vi "Query Active Channel.vi"(8 "error in (no error)":errorcluster, 11 "VISA resource name":refnum<visa-resource-name>) -> (0 "error out":errorcluster, 2 "Active Channel":u16(ring) items=["", "Channel 1", "Channel 2"], 3 "VISA resource name out":refnum<visa-resource-name>)   [LabVIEW 2021, in "Agilent 34420.lvlib"]
doc: "Queries the currently active channel."
uses:
  <instrlib>/Agilent 34420/Agilent 34420.lvlib
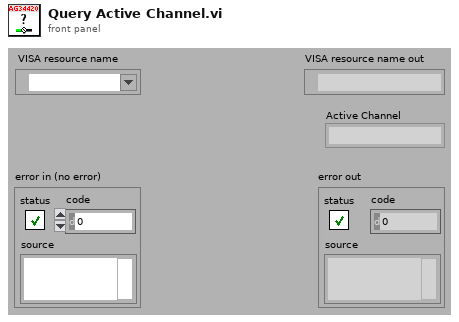
[diagram p1: front panel]
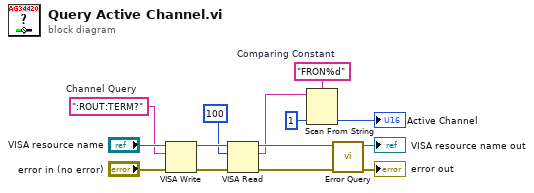
[diagram p0: block diagram]
diagram:
  w3 = "FRON%d"  # Comparing Constant
  w10 = ":ROUT:TERM?"  # Channel Query
  n1 = VISA Write(VISA resource name="VISA resource name", write buffer=w10, error in (no error)="error in (no error)") -> (VISA resource name out=w9:refnum<visa-resource-name>, error out=w8:errorcluster)  [unwired: 1 out]
  n2 = VISA Read(VISA resource name=w9, byte count=u32 100, error in (no error)=w8) -> (VISA resource name out=w7:refnum<visa-resource-name>, read buffer=w4:string, error out=w6:errorcluster)  [unwired: 1 out]
  n3 = Scan From String(format string=w3, input string=w4, default 1=1 ("default value 1")) -> (output 1=→"Active Channel":i32)  [unwired: 2 in, 3 out]
  n4 = call <instrlib>:"Error Query.vi"("error in (no error)"=w6, "VISA resource name"=w7) -> ("error out"=→"error out":errorcluster, "VISA resource name out"=→"VISA resource name out":refnum<visa-resource-name>)  [unwired: 6 in, 2 out]
